vi "Untitled 9.vi"() -> ()   [LabVIEW 2019]
uses:
  Generated_client/RPC Messages/Greeter_req.ctl
  Generated_client/RPC Messages/Greeter_req_req_oneof/Greeter_req_req_oneof.lvclass
  Generated_client/RPC Messages/Greeter_res.ctl
  Generated_client/RPC Messages/Greeter_res_res_oneof/Greeter_res_res_oneof.lvclass
  Generated_client/RPC Messages/Greeter_req_req_oneof/Greeter_req_req_oneof.lvclass/Greeter_req_req_oneof.ctl
  Generated_client/RPC Messages/Greeter_res_res_oneof/Greeter_res_res_oneof.lvclass/Greeter_res_res_oneof.ctl
  Generated_client/Generated_client.lvlib
panel:
  out "OneOfTemplate out":refnum<class "Greeter_res_res_oneof.lvclass">
  out "Get_Val":string
  out "error out 2":errorcluster
  in  "error in (no error)":errorcluster
  out "error out 3":errorcluster
  in  "Set_Val":string
  in  "error in (no error) 2":errorcluster
  out "res_id":i32
  out "error out":errorcluster
  out "Response Data":T1
  in  "Request Data":T2
  in  "address":string
  in  "error in":errorcluster
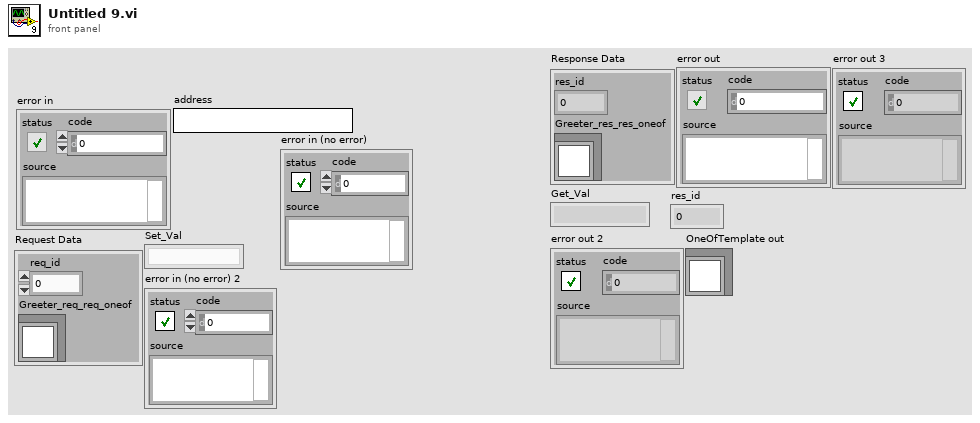
[diagram p1: front panel]
types:
  T1 = typedef "Generated_client.lvlib/Greeter_res.ctl" = cluster{"res_id":i32, "Greeter_res_res_oneof":refnum<class "Greeter_res_res_oneof.lvclass">}
  T2 = typedef "Generated_client.lvlib/Greeter_req.ctl" = cluster{"req_id":i32, "Greeter_req_req_oneof":refnum<class "Greeter_req_req_oneof.lvclass">}
  T3 = typedef "grpc-lvsupport-release.lvlib/grpcId.ctl" = u64
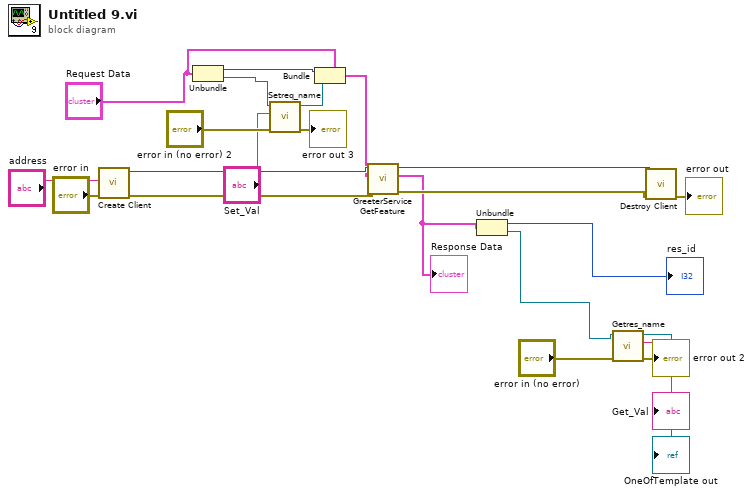
[diagram p0: block diagram]
diagram:
  n1 = call "Create Client.vi"("error in"="error in", "address"="address") -> ("error out"=w20:errorcluster, "gRPC ID Out"=w22:T3)  [unwired: 8 in]
  n2 = Unbundle("Request Data") -> ("req_id"=w15:i32, "Greeter_req_req_oneof"=w10:refnum<class "Greeter_req_req_oneof.lvclass">)
  n3 = call "Setreq_name.vi"("error in (no error)"="error in (no error) 2", "Set_Val"="Set_Val", "OneOfTemplate in"=w10) -> ("error out"=→"error out 3":errorcluster, "OneOfTemplate out"=w9:refnum<class "Greeter_req_req_oneof.lvclass">)  [unwired: 7 in]
  n4 = Bundle(cluster="Request Data", "req_id"=w15, "Greeter_req_req_oneof"=w9) -> (w13:T2)
  n5 = call "GreeterService GetFeature.vi"("error in"=w20, "Request Data"=w13, "gRPC ID"=w22) -> ("error out"=w19:errorcluster, "Response Data"=w11:T1, "gRPC ID out"=w21:T3)  [unwired: 6 in]
  "Response Data" <- w11
  n6 = Unbundle(w11) -> ("res_id"=→"res_id":i32, "Greeter_res_res_oneof"=w5:refnum<class "Greeter_res_res_oneof.lvclass">)
  n7 = call "Getres_name.vi"("error in (no error)"="error in (no error)", "OneOfTemplate in"=w5) -> ("error out"=→"error out 2":errorcluster, "Get_Val"=→"Get_Val":string, "OneOfTemplate out"=→"OneOfTemplate out":refnum<class "Greeter_res_res_oneof.lvclass">)  [unwired: 7 in]
  n8 = call "Destroy Client.vi"("error in"=w19, "gRPC ID"=w21) -> ("error out"=→"error out":errorcluster)  [unwired: 9 in]
